vi "FTT subpanel Query.vi"(8 "error in (no error)":errorcluster, 11 "Cluster":T10 {"Main"."VISA"."flow control" items=["None", "XON/XOFF", "RTS/CTS", "XON/XOFF & RTS/CTS", "DTR/DSR", "XON/XOFF & DTR/DSR"]; "Main"."VISA"."stop bits" items=["1.0"=10, "1.5"=15, "2.0"=20]; "DB Dispaly"."StartTime" format="%<%Y/%m/%d %H:%M>T"; "DB Dispaly"."EndTime" format="%<%Y/%m/%d %H:%M>T"}) -> (0 "error out":errorcluster, 3 "DB Dispaly":T9 {"StartTime" format="%<%Y/%m/%d %H:%M>T"; "EndTime" format="%<%Y/%m/%d %H:%M>T"})   [LabVIEW 2014]
uses:
  <vilib>/addons/database/NI_Database_API.lvlib
  <vilib>/addons/database/_DB Variant To Data/Database Variant To Data.xnode
  Type'def/DB Query.ctl
  Type'def/UPH Config.ctl
  VISA/Ctr/VISA Ctr.ctl
  Type'def/Main Ctr Ref.ctl
  Type'def/User Login.ctl
  Database/Ctr/Constr.ctl
  <vilib>/addons/database/Connection.llb/Conn ObjectReference.ctl
  Database/Ctr/Conneect State.ctl
  Type'def/MainCtr.ctl
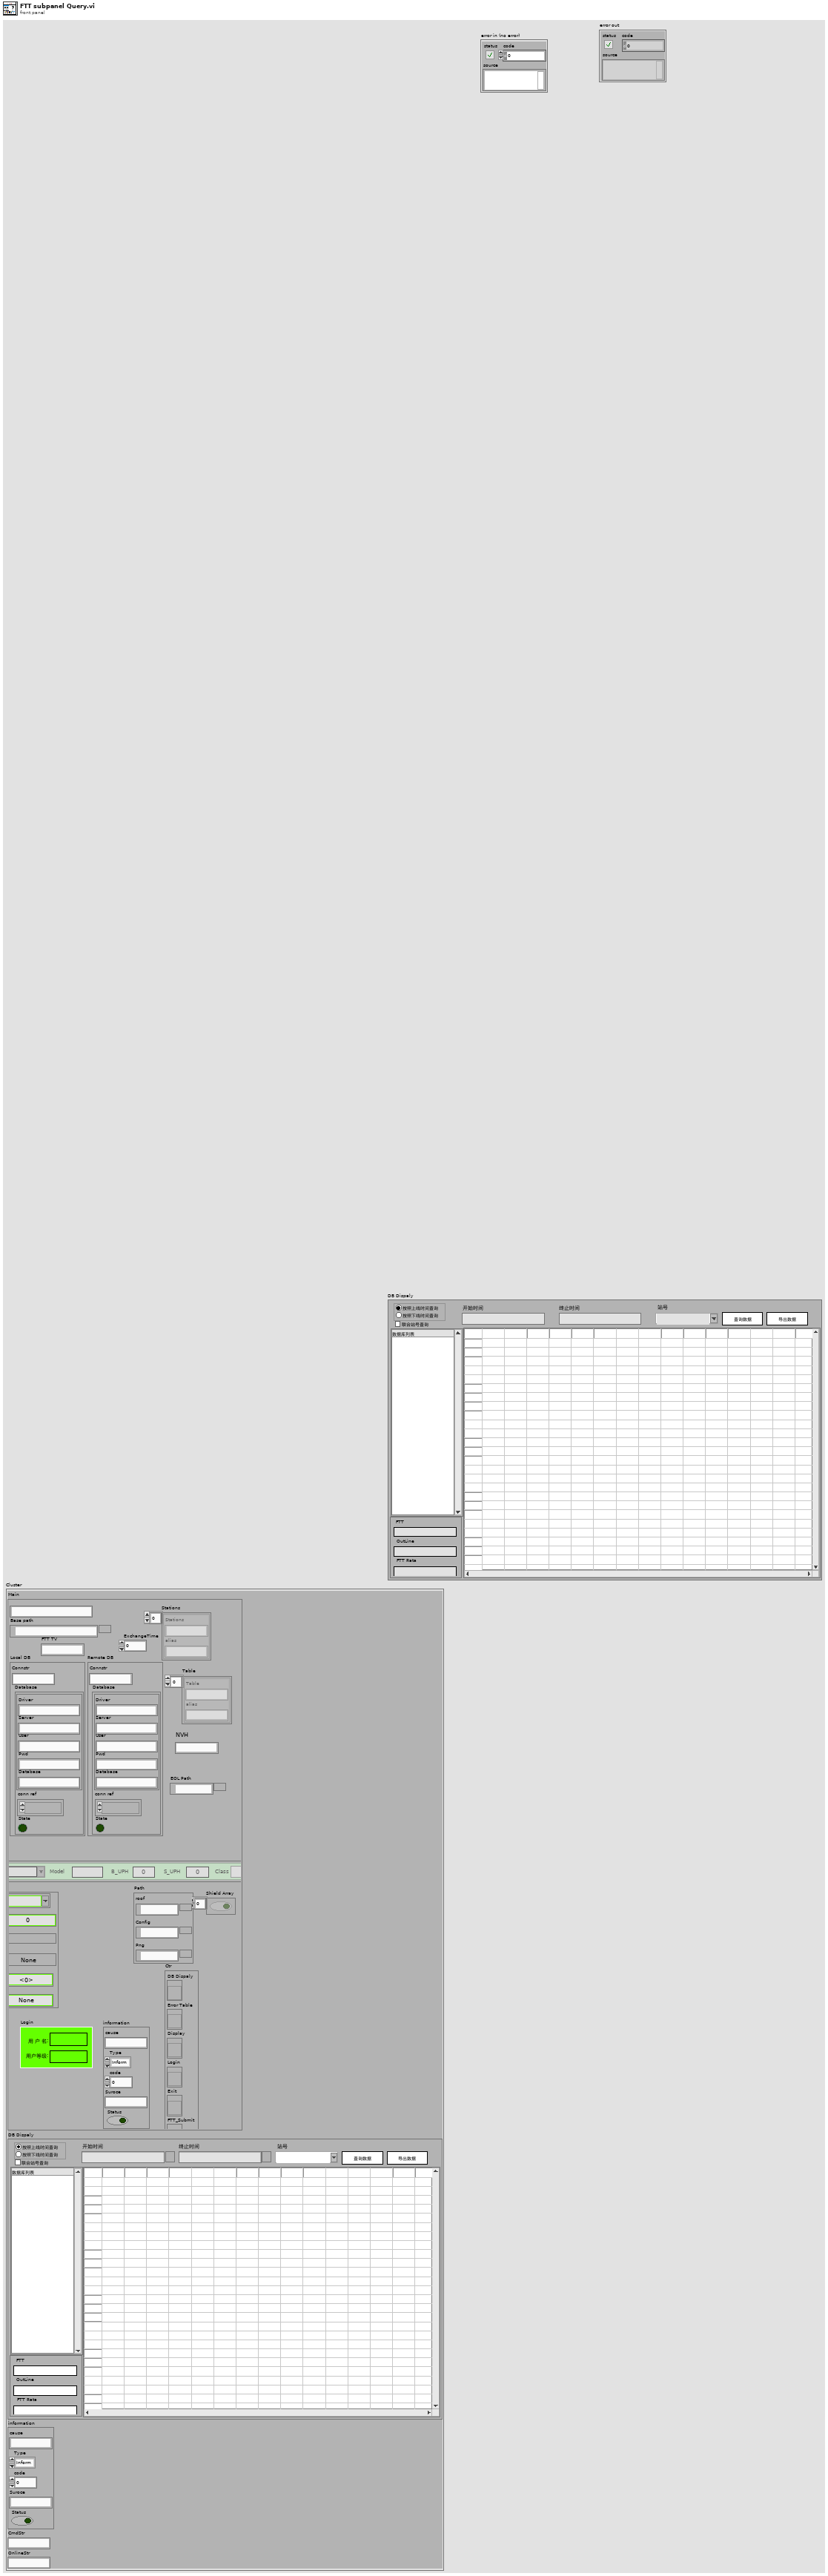
[diagram p1: front panel]
types:
  T1 = typedef "MainCtr.ctl" = cluster{"Tite":string, "Base path":path, "Table":cluster{"Table":string, "alias":string}[], "Stations":cluster{"Stations":string, "alias":string}[], "Shield Array":bool[], "UPHs":T2[], "VISA":T3, "Path":cluster{"roof":path, "Config":path, "Png":path}, "Ctr":T4, "Login":T5, "information":cluster{"cause":string, "Type":enum16{"Inform", "Warning", "Alarm"}, "code":i32, "Suroce":string, "Status":bool}, "Local DB":cluster{"Connstr":string, "Database":T6}, "Remote DB":cluster{"Connstr":string, "Database":T6}, "FTT TV":string, "ExchangeTime":i32, "NVH":string, "EOL Path":path}
  T2 = typedef "UPH Config.ctl" = cluster{"Line_No":string, "Model":string, "B_UPH ":i16, "S_UPH  ":i16, "Class":enum16{"Big", "Small"}}
  T3 = typedef "VISA Ctr.ctl" = cluster{"VISA":refnum<visa-resource-name>, "baud rate":u32, "data bits":u16, "parity":enum16{"None", "Odd", "Even", "Mark", "Space"}, "stop bits":u16, "flow control":u16}
  T4 = typedef "Main Ctr Ref.ctl" = cluster{"DB Dispaly":refnum<vi>, "Error Table":refnum<vi>, "Display":refnum<vi>, "Login":refnum<vi>, "Exit":refnum<vi>, "FTT_Submit":refnum<vi>}
  T5 = typedef "User Login.ctl" = cluster{"User":string, "Grade":string}
  T6 = typedef "Conneect State.ctl" = cluster{"Constr":T7, "conn ref":T8, "State":bool}
  T7 = typedef "Constr.ctl" = cluster{"Driver":string, "Server":string, "User":string, "Pwd":string, "Database":string}
  T8 = typedef "NI_Database_API.lvlib/Conn ObjectReference.ctl" = refnum<k1>
  T9 = typedef "DB Query.ctl" = cluster{"Export":bool, "Query":bool, "Station.No":string, "EndTime":timestamp, "StartTime":timestamp, "FTT":cluster{"FTT":string, "OutLine":string, "FTT Rata":string}, "TableName":string, "List":string[][], "Station":bool, "QTime":enum32{"Online", "Outline"}}
  T10 = cluster{"Main ":T1, "DB Dispaly":T9, "information":cluster{"cause":string, "Type":enum16{"Inform", "Warning", "Alarm"}, "code":i32, "Suroce":string, "Status":bool}, "CmdStr":string, "OnlineStr":string}
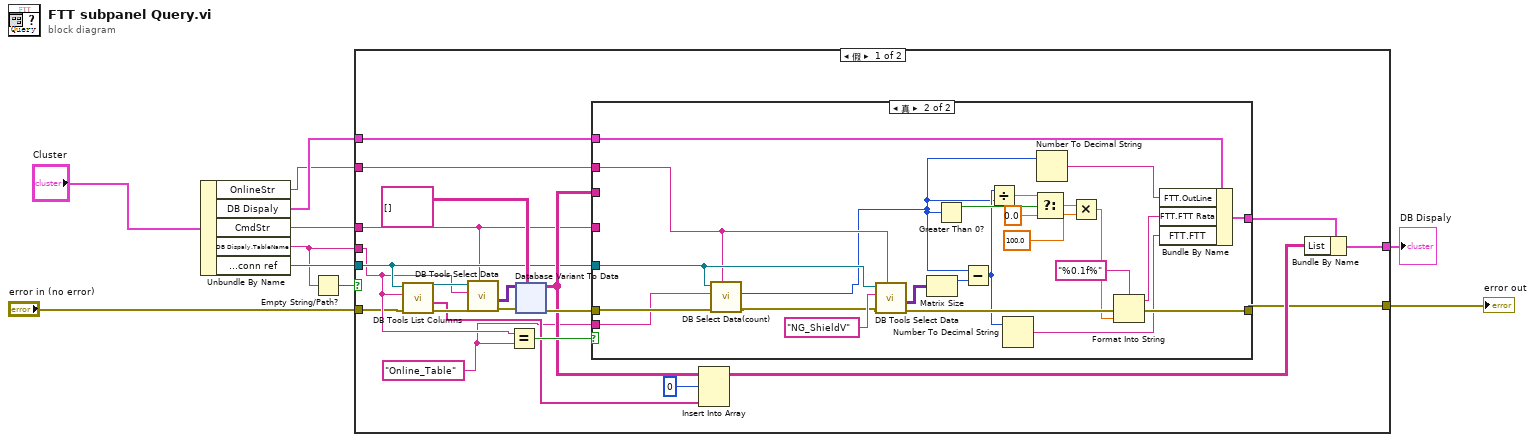
[diagram p0: block diagram]
diagram:
  n1 = Unbundle By Name("Cluster") -> ("OnlineStr"=w1:string, "DB Dispaly"=w5:T9, "CmdStr"=w6:string, "DB Dispaly.TableName"=w8:string, "Main.Local DB.Database.conn ref"=w9:T8)
  n2 = Empty String/Path?(string/path=w8) -> (empty?=w7:bool)
  n3 = case shown="假" w7 {
    tunnel: [w19 w103] -> w10
    tunnel: w9 -> [w18 _]
    tunnel: w8 -> [w17 _]
    tunnel: w6 -> [w16 _]
    tunnel: w5 -> [w15 w102]
    tunnel: [w14 w102] -> w3
    tunnel: "error in (no error)" -> [w13 w103]
    tunnel: w1 -> [w11 _]
    frame False {
      w12 = "Online_Table"
      n4 = call <vilib>:"DB Tools List Columns.vi"("error in (no error)"=w13, "table"=w17, "connection reference"=w18) -> ("error out"=w24:errorcluster, "columns"=w22:string[], "connection reference out"=w25:T8)  [unwired: 1 in, 1 out]
      n5 = call <vilib>:"DB Tools Select Data.vi"("condition"=w16, "error in (no error)"=w24, "table"=w17, "connection reference"=w25) -> ("error out"=w31:errorcluster, "data"=w30:variant[][])  [unwired: 2 in, 1 out]
      n6 = Equal?(x=w17, y=w12) -> (x = y?=w28:bool)
      n7 = xnode "Database Variant To Data"("database variant"=w30, "error in (no error)"=w31, "type"=string[][] []) -> ("data"=w23:string[][], "error out"=w27:errorcluster)
      n8 = case shown="真" w28 {
        tunnel: w27 -> [w33 w39]
        tunnel: w18 -> [_ w38]
        tunnel: w16 -> [_ _]
        tunnel: w23 -> [_ _]
        tunnel: [w33 w46] -> w19
        tunnel: [w32 w41] -> w26
        tunnel: w15 -> [w32 w40]
        tunnel: w12 -> [_ w37]
        tunnel: w11 -> [_ w36]
        frame False {
        }
        frame True {
          n9 = call "DB Select Data(count).vi"("condition"=w36, "error in (no error)"=w39, "table"=w37, "connection reference"=w38) -> ("error out"=w35:errorcluster, "Count"=w34:i32)  [unwired: 5 in, 1 out]
          n10 = call <vilib>:"DB Tools Select Data.vi"("condition"=w36, "error in (no error)"=w35, "table"="NG_ShieldV", "connection reference"=w38) -> ("error out"=w49:errorcluster, "data"=w56:variant[][])  [unwired: 2 in, 1 out]
          n11 = Matrix Size(0:w56) -> (1:w55:i32)  [unwired: 1 out]
          n12 = Greater Than 0?(x=w34) -> (x > 0?=w53:bool)
          n13 = Subtract(x=w34, y=w55) -> (x-y=w44:i32)
          n14 = Divide(x=w44, y=w34) -> (x/y=w54:dbl)
          n15 = Number To Decimal String(number=w44) -> (decimal integer string=w42:string)  [unwired: 1 in]
          n16 = Select(t=w54, s=w53, f=0.0) -> (s? t:f=w51:dbl)
          n17 = Number To Decimal String(number=w34) -> (decimal integer string=w45:string)  [unwired: 1 in]
          n18 = Multiply(x=w51, y=100.0) -> (x*y=w48:dbl)
          n19 = Format Into String(format string="%0.1f%", error in=w49, w48) -> (resulting string=w43:string, error out=w46:errorcluster)  [unwired: 1 in]
          n20 = Bundle By Name(cluster=w40, "FTT.OutLine"=w45, "FTT.FTT Rata"=w43, "FTT.FTT"=w42) -> (w41:T9)
        }
      }
      n21 = Insert Into Array(array=w23, index (row)=0, new element=w22) -> (w20:string[][])  [unwired: 1 in]
      n22 = Bundle By Name(cluster=w26, "List"=w20) -> (w14:T9)
    }
    frame True {
    }
  }
  "error out" <- w10
  "DB Dispaly" <- w3
